vi "Receive PF Commands.vi"(8 "error in (no error)":errorcluster, 9 "Setpoint":dbl, 10 "Run":bool, 11 "Test in":refnum<class "Test.lvclass">) -> (0 "error out":errorcluster, 3 "Test out":refnum<class "Test.lvclass">)   [LabVIEW 2019, in "Test.lvlib" / "Test.lvclass"]
uses:
  Test.lvclass
  C:/Program Files (x86)/National Instruments/LabVIEW 2019/vi.lib/ActorFramework/Actor/Actor.lvclass
  <vilib>/ActorFramework/Actor/Actor.lvclass/Actor.ctl
  <vilib>/ActorFramework/Message Enqueuer/Message Enqueuer.lvclass/Message Enqueuer.ctl
  Test.lvclass/Test.ctl
  Test Messages/Update Set Temp Msg/Update Set Temp Msg.lvclass/Update Set Temp Msg.ctl
  Power Supply/Power Supply Messages/PF2PS Msg/PF2PS Msg.lvclass/PF2PS Msg.ctl
  <vilib>/ActorFramework/Message Enqueuer/Init from Existing Queue.vi
  <vilib>/ActorFramework/Message Enqueuer/Enqueue.vi
  Test Messages/Update Set Temp Msg/Update Set Temp Msg.lvclass
  C:/Program Files (x86)/National Instruments/LabVIEW 2019/vi.lib/ActorFramework/Message/Message.lvclass
  Power Supply/Power Supply Messages/PF2PS Msg/PF2PS Msg.lvclass
  <vilib>/ActorFramework/Message Priority Queue/Priority Enqueue.vi
  <vilib>/ActorFramework/Message Enqueuer/Message Enqueuer.lvclass
  Cobra RT AF/Cobra RT/Cobra RT Messages/Receive Setpoint Msg/Receive Setpoint Msg.lvclass
  <vilib>/ActorFramework/Actor/Actor.lvclass
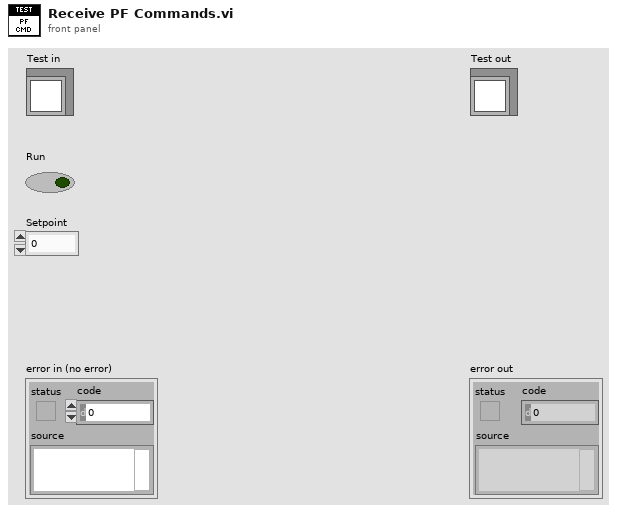
[diagram p1: front panel]
types:
  T1 = map{string, cluster{"Selected Heads":string, "Instrument":refnum<class "Message Enqueuer.lvclass">, "Platform":refnum<class "Message Enqueuer.lvclass">}}
  T2 = cluster{"Selected Heads":string, "Instrument":refnum<class "Message Enqueuer.lvclass">, "Platform":refnum<class "Message Enqueuer.lvclass">}
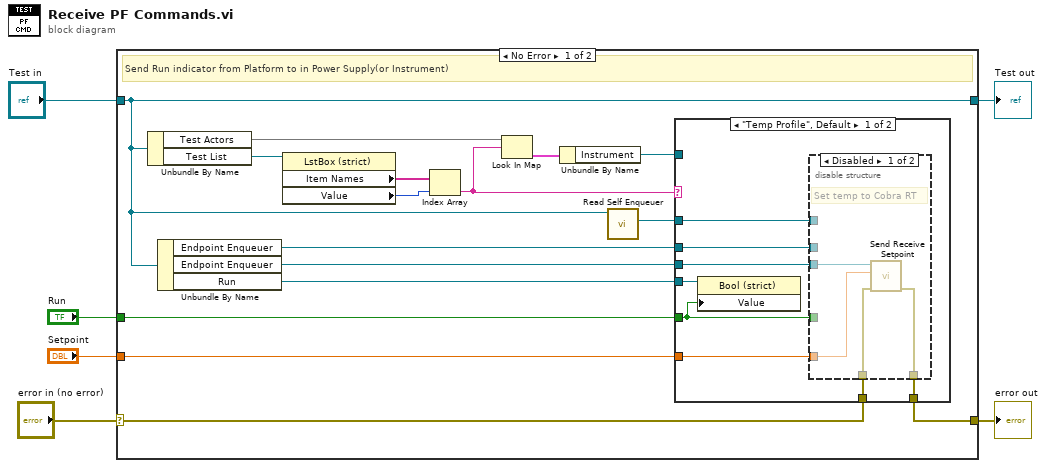
[diagram p0: block diagram]
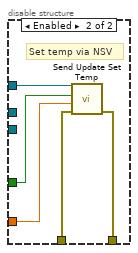
[diagram p2: hidden frame]
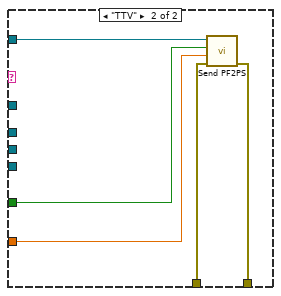
[diagram p3: hidden frame]
diagram:
  n1 = case shown="No Error" "error in (no error)" {
    selector: "error in (no error)" -> [w14 w46]
    tunnel: [w11 w46] -> w5
    tunnel: [w8 w45] -> w4
    tunnel: "Test in" -> [w8 w45]
    tunnel: "Run" -> [w10 _]
    tunnel: "Setpoint" -> [w15 _]
    frame No Error {
      # "Send Run indicator from Platform to in Power Supply(or Instrument)"
      n2 = Unbundle By Name(w8) -> ("Test Actors"=w18:T1, "Test List"=w22:refnum<vi>)
      n3 = Unbundle By Name(w8) -> ("Endpoint Enqueuer"=w13:refnum<class "Message Enqueuer.lvclass">, "Endpoint Enqueuer"=w12:refnum<class "Message Enqueuer.lvclass">, "Run"=w7:refnum<vi>)
      n4 = property class="LstBox (strict)"(reference=w22) -> ("Item Names"=w21:string[], "Value"=w20:i32)  [unwired: 1 in, 2 out]
      n5 = Index Array(array=w21, index=w20) -> (element=w17:string)
      n6 = Look In Map(map=w18, key=w17) -> (value=w19:T2)  [unwired: 1 in, 1 out]
      n7 = Unbundle By Name(w19) -> ("Instrument"=w16:refnum<class "Message Enqueuer.lvclass">)
      n8 = call <vilib>:"Read Self Enqueuer.vi"("Actor"=w8) -> ("Self Enqueuer"=w9:refnum<class "Message Enqueuer.lvclass">)  [unwired: 10 in]
      n9 = case shown="\"Temp Profile\", Default" w17 {
        tunnel: w16 -> [_ w44]
        tunnel: w10 -> [w23 w43]
        tunnel: w15 -> [w29 w42]
        tunnel: w14 -> [w27 w41]
        tunnel: w12 -> [w30 _]
        tunnel: w13 -> [w28 _]
        tunnel: [w26 w40] -> w11
        tunnel: w9 -> [w25 _]
        tunnel: w7 -> [w24 _]
        frame "Temp Profile", Default {
          n10 = property class="Bool (strict)"(reference=w24, "Value"=w23) -> ()  [unwired: 1 in, 2 out]
          n11 = disable-structure shown="Disabled" {
            disable-tunnel: w30 -> [w34 _]
            disable-tunnel: w29 -> [w33 w36]
            disable-tunnel: w23 -> [_ w37]
            disable-tunnel: w28 -> [_ _]
            disable-tunnel: w27 -> [w32 w39]
            disable-tunnel: [w31 w38] -> w26
            disable-tunnel: w25 -> [_ w35]
            frame Disabled {
              # "Set temp to Cobra RT"
              n12 = call "Send Receive Setpoint.vi"("error in (no error)"=w32, "Set Temp"=w33, "Message Enqueuer"=w34) -> ("error out"=w31:errorcluster)  [unwired: 7 in, 1 out]
            }
            frame Enabled {
              # "Set temp via NSV"
              n13 = call "Send Update Set Temp.vi"("error in (no error)"=w39, "Setpoint"=w36, "Run"=w37, "Message Enqueuer"=w35) -> ("error out"=w38:errorcluster)  [unwired: 6 in, 1 out]
            }
          }
        }
        frame "TTV" {
          n14 = call "Send PF2PS.vi"("error in (no error)"=w41, "Setpoint"=w42, "Run"=w43, "Message Enqueuer"=w44) -> ("error out"=w40:errorcluster)  [unwired: 6 in, 1 out]
        }
      }
    }
    frame Error {
    }
  }
  "error out" <- w5
  "Test out" <- w4
